vi "RecordTrig_DerotatorControl.vi"() -> ()   [LabVIEW 2021]
uses:
  <vilib>/DAQmx/write.llb/DAQmx Write (Digital Bool 1Line 1Point).vi
  <vilib>/DAQmx/create/channels.llb/DAQmx Create Channel (DO-Digital Output).vi
  <vilib>/DAQmx/miscellaneous.llb/DAQmx Fill In Error Info.vi
panel:
  in  "pulse wait":u32=50
  in  "Move Derotator":bool
  in  "Direction":bool
  in  "stop":bool
  in  "Record!":bool
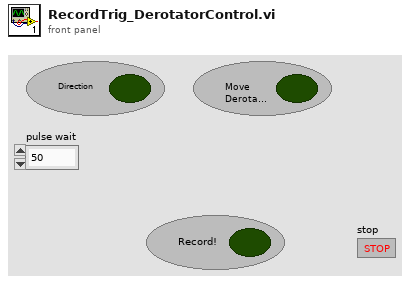
[diagram p1: front panel]
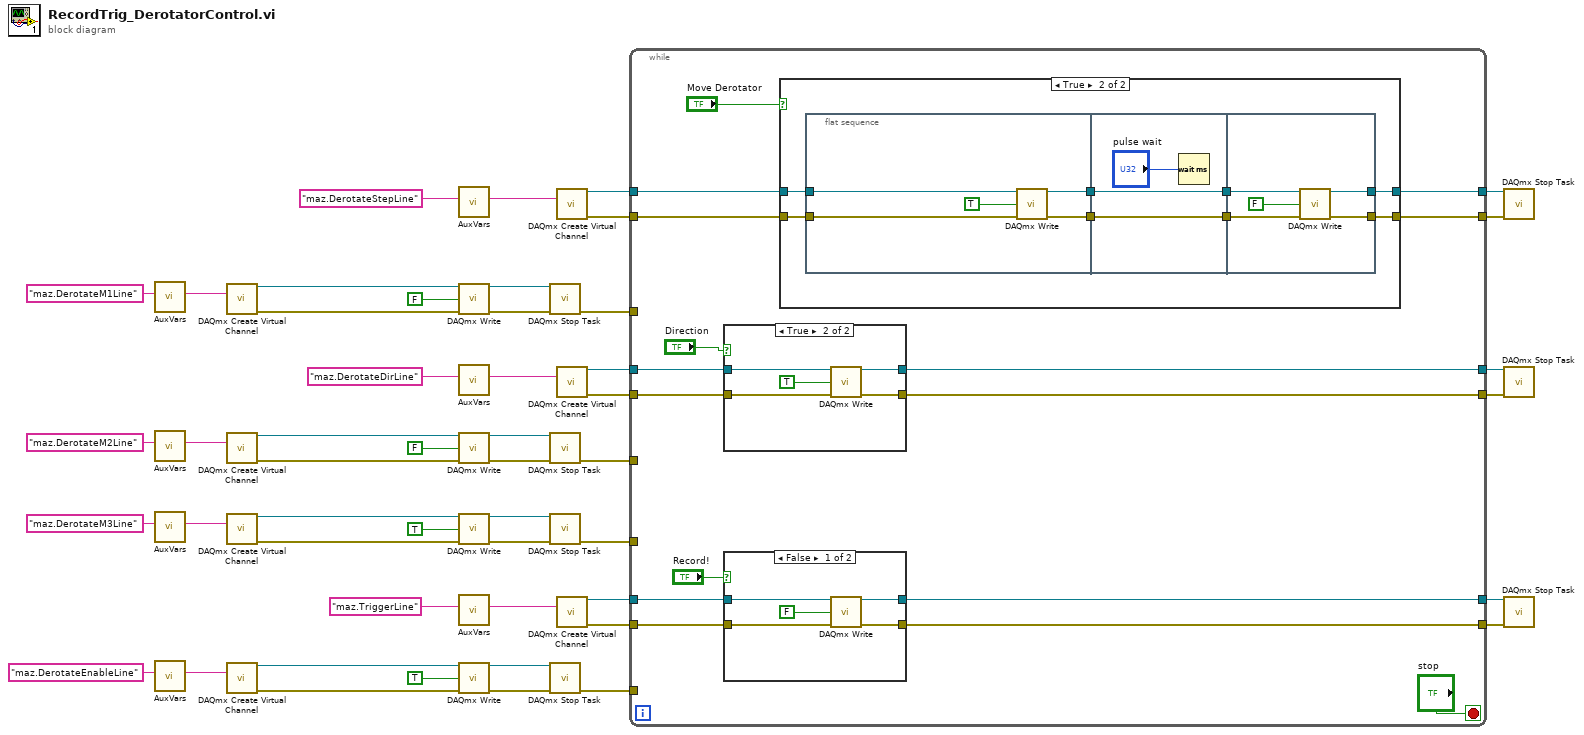
[diagram p0: block diagram]
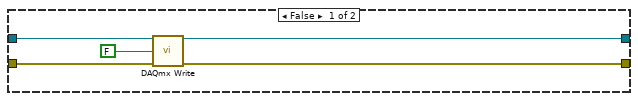
[diagram p2: hidden frame]
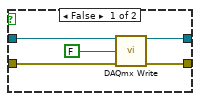
[diagram p3: hidden frame]
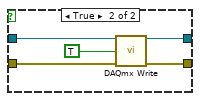
[diagram p4: hidden frame]
diagram:
  n1 = call "AuxVars.vi"("key"="maz.DerotateM1Line") -> ("value"=w25:string)  [unwired: 9 in, 1 out]
  n2 = call "AuxVars.vi"("key"="maz.DerotateM2Line") -> ("value"=w18:string)  [unwired: 9 in, 1 out]
  n3 = call "AuxVars.vi"("key"="maz.DerotateM3Line") -> ("value"=w11:string)  [unwired: 9 in, 1 out]
  n4 = call "AuxVars.vi"("key"="maz.DerotateEnableLine") -> ("value"=w40:string)  [unwired: 9 in, 1 out]
  n5 = call-poly <vilib>:"DAQmx Create Virtual Channel.vi"("lines"=w25) -> ("task out"=w22:refnum<k21>, "error out"=w19:errorcluster)  [unwired: 13 in]
  n6 = call-poly <vilib>:"DAQmx Create Virtual Channel.vi"("lines"=w18) -> ("task out"=w15:refnum<k21>, "error out"=w12:errorcluster)  [unwired: 13 in]
  n7 = call-poly <vilib>:"DAQmx Create Virtual Channel.vi"("lines"=w11) -> ("task out"=w8:refnum<k21>, "error out"=w5:errorcluster)  [unwired: 13 in]
  n8 = call-poly <vilib>:"DAQmx Create Virtual Channel.vi"("lines"=w40) -> ("task out"=w29:refnum<k21>, "error out"=w26:errorcluster)  [unwired: 13 in]
  n9 = call "AuxVars.vi"("key"="maz.DerotateStepLine") -> ("value"=w42:string)  [unwired: 9 in, 1 out]
  n10 = call-poly <vilib>:"DAQmx Write.vi"("task/channels in"=w22, "data"=FALSE, "error in"=w19) -> ("task out"=w21:refnum<k21>, "error out"=w20:errorcluster)  [unwired: 10 in, 1 out]
  n11 = call "AuxVars.vi"("key"="maz.DerotateDirLine") -> ("value"=w44:string)  [unwired: 9 in, 1 out]
  n12 = call-poly <vilib>:"DAQmx Write.vi"("task/channels in"=w15, "data"=FALSE, "error in"=w12) -> ("task out"=w14:refnum<k21>, "error out"=w13:errorcluster)  [unwired: 10 in, 1 out]
  n13 = call-poly <vilib>:"DAQmx Write.vi"("task/channels in"=w8, "data"=TRUE, "error in"=w5) -> ("task out"=w7:refnum<k21>, "error out"=w6:errorcluster)  [unwired: 10 in, 1 out]
  n14 = call "AuxVars.vi"("key"="maz.TriggerLine") -> ("value"=w50:string)  [unwired: 9 in, 1 out]
  n15 = call-poly <vilib>:"DAQmx Write.vi"("task/channels in"=w29, "data"=TRUE, "error in"=w26) -> ("task out"=w28:refnum<k21>, "error out"=w27:errorcluster)  [unwired: 10 in, 1 out]
  n16 = call <vilib>:"DAQmx Stop Task.vi"("task/channels in"=w21, "error in"=w20) -> ("error out"=w3:errorcluster)  [unwired: 12 in, 1 out]
  n17 = call <vilib>:"DAQmx Stop Task.vi"("task/channels in"=w14, "error in"=w13) -> ("error out"=w2:errorcluster)  [unwired: 12 in, 1 out]
  n18 = call <vilib>:"DAQmx Stop Task.vi"("task/channels in"=w7, "error in"=w6) -> ("error out"=w1:errorcluster)  [unwired: 12 in, 1 out]
  n19 = call <vilib>:"DAQmx Stop Task.vi"("task/channels in"=w28, "error in"=w27) -> ("error out"=w4:errorcluster)  [unwired: 12 in, 1 out]
  n20 = call-poly <vilib>:"DAQmx Create Virtual Channel.vi"("lines"=w42) -> ("task out"=w38:refnum<k21>, "error out"=w37:errorcluster)  [unwired: 13 in]
  n21 = call-poly <vilib>:"DAQmx Create Virtual Channel.vi"("lines"=w44) -> ("task out"=w34:refnum<k21>, "error out"=w33:errorcluster)  [unwired: 13 in]
  n22 = call-poly <vilib>:"DAQmx Create Virtual Channel.vi"("lines"=w50) -> ("task out"=w48:refnum<k21>, "error out"=w47:errorcluster)  [unwired: 13 in]
  n23 = while {
    tunnel: w48 -> [w66]
    tunnel: w47 -> [w65]
    tunnel: [w64] -> w46
    tunnel: [w63] -> w45
    tunnel: w38 -> [w58]
    tunnel: w37 -> [w57]
    tunnel: [w56] -> w36
    tunnel: [w55] -> w35
    tunnel: w34 -> [w54]
    tunnel: w33 -> [w53]
    tunnel: [w52] -> w32
    tunnel: [w51] -> w31
    tunnel: w4 -> [_]
    tunnel: w3 -> [_]
    tunnel: w2 -> [_]
    tunnel: w1 -> [_]
    stop <- "stop" stop-if-true
    n24 = case shown="True" "Direction" {
      tunnel: w54 -> [w96 w102]
      tunnel: w53 -> [w95 w101]
      tunnel: [w94 w100] -> w51
      tunnel: [w93 w99] -> w52
      frame False {
        n25 = call-poly <vilib>:"DAQmx Write.vi"("task/channels in"=w96, "data"=FALSE, "error in"=w95) -> ("task out"=w94:refnum<k21>, "error out"=w93:errorcluster)  [unwired: 10 in, 1 out]
      }
      frame True {
        n26 = call-poly <vilib>:"DAQmx Write.vi"("task/channels in"=w102, "data"=TRUE, "error in"=w101) -> ("task out"=w100:refnum<k21>, "error out"=w99:errorcluster)  [unwired: 10 in, 1 out]
      }
    }
    n27 = case shown="False" "Record!" {
      tunnel: w66 -> [w106 w112]
      tunnel: w65 -> [w105 w111]
      tunnel: [w104 w110] -> w64
      tunnel: [w103 w109] -> w63
      frame False {
        n28 = call-poly <vilib>:"DAQmx Write.vi"("task/channels in"=w106, "data"=FALSE, "error in"=w105) -> ("task out"=w104:refnum<k21>, "error out"=w103:errorcluster)  [unwired: 10 in, 1 out]
      }
      frame True {
        n29 = call-poly <vilib>:"DAQmx Write.vi"("task/channels in"=w112, "data"=TRUE, "error in"=w111) -> ("task out"=w110:refnum<k21>, "error out"=w109:errorcluster)  [unwired: 10 in, 1 out]
      }
    }
    n30 = case shown="True" "Move Derotator" {
      tunnel: w58 -> [w70 w79]
      tunnel: w57 -> [w69 w78]
      tunnel: [w68 w72] -> w55
      tunnel: [w67 w73] -> w56
      frame False {
        n31 = call-poly <vilib>:"DAQmx Write.vi"("task/channels in"=w70, "data"=FALSE, "error in"=w69) -> ("task out"=w68:refnum<k21>, "error out"=w67:errorcluster)  [unwired: 10 in, 1 out]
      }
      frame True {
        n32 = flat-sequence {
          tunnel: w79 -> [w84]
          tunnel: w78 -> [w83]
          tunnel: [w82] -> w77
          tunnel: [w80] -> w75
          tunnel: w77 -> [w87]
          tunnel: [w87] -> w76
          tunnel: w75 -> [w85]
          tunnel: [w85] -> w74
          tunnel: w76 -> [w92]
          tunnel: w74 -> [w90]
          tunnel: [w89] -> w73
          tunnel: [w88] -> w72
          frame #0 {
            n33 = call-poly <vilib>:"DAQmx Write.vi"("task/channels in"=w84, "data"=TRUE, "error in"=w83) -> ("task out"=w82:refnum<k21>, "error out"=w80:errorcluster)  [unwired: 10 in, 1 out]
          }
          frame #1 {
            n34 = Wait (ms)(milliseconds to wait="pulse wait") -> ()  [unwired: 1 out]
          }
          frame #2 {
            n35 = call-poly <vilib>:"DAQmx Write.vi"("task/channels in"=w92, "data"=FALSE, "error in"=w90) -> ("task out"=w88:refnum<k21>, "error out"=w89:errorcluster)  [unwired: 10 in, 1 out]
          }
        }
      }
    }
  }
  n36 = call <vilib>:"DAQmx Stop Task.vi"("task/channels in"=w35, "error in"=w36) -> ()  [unwired: 12 in, 2 out]
  n37 = call <vilib>:"DAQmx Stop Task.vi"("task/channels in"=w31, "error in"=w32) -> ()  [unwired: 12 in, 2 out]
  n38 = call <vilib>:"DAQmx Stop Task.vi"("task/channels in"=w46, "error in"=w45) -> ()  [unwired: 12 in, 2 out]
